vi "MGI Set Table Scrollbar.vi"(10 "Error In":errorcluster, 11 "Listbox Reference In":refnum<vi>) -> (2 "Error Out":errorcluster, 3 "Listbox Reference Out":refnum<vi>)   [LabVIEW 2020]
doc: "Show or hide the specified Table's horizontal and vertical scrollbars based on the table's contents. This VI will also set the scrollbar position as necessary to ensure that some of the table's contents is displayed.\n\nAuthored by Shawn Walpole\nsupport@mooregoodideas.com\nwww.mooregoodideas.com\n\nCopyright (c) 2010, Moore Good Ideas, Inc.\n\nAll rights reserved.\n\nRedistribution and use in source and binary forms, with or without modification, are permitted provided that the following conditions are met:\n\n * Redistributions of source code must retain the above copyright notice, this list of conditions and the following disclaimer.\n * Redistributions in binary form must reproduce the above copyright notice, this list of conditions and the following disclaimer in the documentation and/or other materials provided with the distribution.\n * Neither the name of Moore Good Ideas, Inc. nor the names of its contributors may be used to endorse or promote products derived from this software without specific prior written permission.\n\nTHIS SOFTWARE IS PROVIDED BY THE COPYRIGHT HOLDERS AND CONTRIBUTORS \"AS IS\" AND ANY EXPRESS OR IMPLIED WARRANTIES, INCLUDING, BUT NOT LIMITED TO, THE IMPLIED WARRANTIES OF MERCHANTABILITY AND FITNESS FOR A PARTICULAR PURPOSE ARE DISCLAIMED. IN NO EVENT SHALL THE COPYRIGHT OWNER OR CONTRIBUTORS BE LIABLE FOR ANY DIRECT, INDIRECT, INCIDENTAL, SPECIAL, EXEMPLARY, OR CONSEQUENTIAL DAMAGES (INCLUDING, BUT NOT LIMITED TO, PROCUREMENT OF SUBSTITUTE GOODS OR SERVICES; LOSS OF USE, DATA, OR PROFITS; OR BUSINESS INTERRUPTION) HOWEVER CAUSED AND ON ANY THEORY OF LIABILITY, WHETHER IN CONTRACT, STRICT LIABILITY, OR TORT (INCLUDING NEGLIGENCE OR OTHERWISE) ARISING IN ANY WAY OUT OF THE USE OF THIS SOFTWARE, EVEN IF ADVISED OF THE POSSIBILITY OF SUCH DAMAGE."
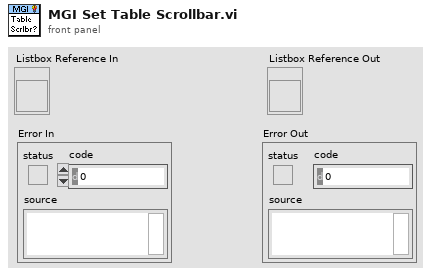
[diagram p1: front panel]
types:
  T1 = typedef "LVRowAndColumnUnsignedTypeDef.ctl" = cluster{"Row":u32, "Column":u32}
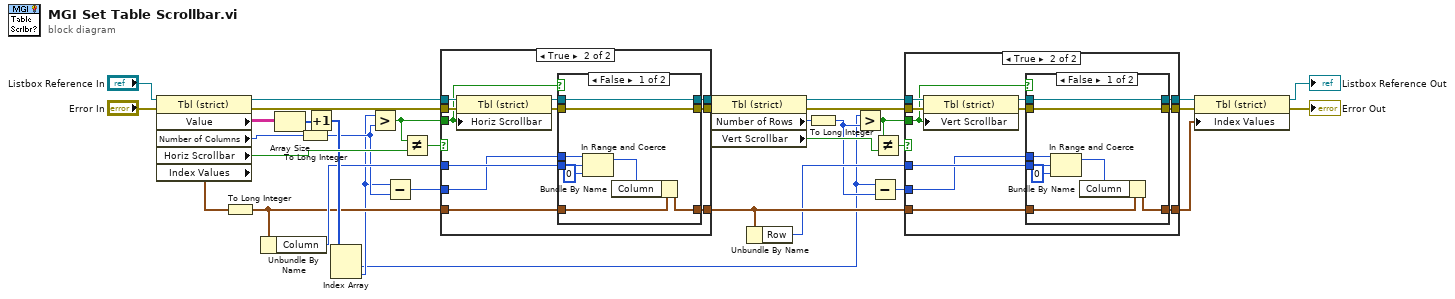
[diagram p0: block diagram]
diagram:
  n1 = property class="Tbl (strict)"(reference="Listbox Reference In", error in="Error In") -> (reference out=w35:refnum<vi>, error out=w27:errorcluster, "Value"=w33:string[][], "Number of Columns"=w26:u32, "Horiz Scrollbar"=w31:bool, "Index Values"=w6:T1)
  n2 = To Long Integer(number=w6) -> (32bit integer=w5:cluster{"Row":i32, "Column":i32})
  n3 = Unbundle By Name(w5) -> ("Column"=w23:i32)
  n4 = Array Size(array=w33) -> (size(s)=w32:i32[])
  n5 = To Long Integer(number=w26) -> (32bit integer=w7:i32)
  n6 = Increment(x=w32) -> (x+1=w24:i32[])
  n7 = Index Array(array=w24) -> (element #1=w1:i32, element #2=w2:i32)  [unwired: 2 in]
  n8 = Greater?(x=w2, y=w7) -> (0:w30:bool)
  n9 = Subtract(x=w2, y=w7) -> (x-y=w25:i32)
  n10 = Not Equal?(x=w30, y=w31) -> (x != y?=w29:bool)
  n11 = case shown="True" w29 {
    tunnel: w35 -> [w38 w49]
    tunnel: w30 -> [_ w43]
    tunnel: [w38 w45] -> w18
    tunnel: w27 -> [w37 w48]
    tunnel: [w37 w44] -> w16
    tunnel: w23 -> [_ w42]
    tunnel: w25 -> [_ w41]
    tunnel: w5 -> [w36 w40]
    tunnel: [w36 w39] -> w20
    frame False {
    }
    frame True {
      n12 = property class="Tbl (strict)"(reference=w49, error in=w48, "Horiz Scrollbar"=w43) -> (reference out=w47:refnum<vi>, error out=w46:errorcluster)
      n13 = case shown="False" w43 {
        tunnel: w47 -> [w52 w60]
        tunnel: w46 -> [w53 w59]
        tunnel: [w52 w60] -> w45
        tunnel: [w53 w59] -> w44
        tunnel: w42 -> [w57 _]
        tunnel: w41 -> [w55 _]
        tunnel: w40 -> [w54 w58]
        tunnel: [w50 w58] -> w39
        frame False {
          n14 = In Range and Coerce(upper limit=w55, x=w57, lower limit=0) -> (coerced(x)=w51:i32)  [unwired: 1 out]
          n15 = Bundle By Name(cluster=w54, "Column"=w51) -> (w50:cluster{"Row":i32, "Column":i32})
        }
        frame True {
        }
      }
    }
  }
  n16 = property class="Tbl (strict)"(reference=w18, error in=w16) -> (reference out=w19:refnum<vi>, error out=w17:errorcluster, "Number of Rows"=w4:u32, "Vert Scrollbar"=w14:bool)
  n17 = Unbundle By Name(w20) -> ("Row"=w15:i32)
  n18 = To Long Integer(number=w4) -> (32bit integer=w3:i32)
  n19 = Greater?(x=w1, y=w3) -> (0:w13:bool)
  n20 = Subtract(x=w1, y=w3) -> (x-y=w21:i32)
  n21 = Not Equal?(x=w13, y=w14) -> (x != y?=w22:bool)
  n22 = case shown="True" w22 {
    tunnel: w19 -> [w63 w74]
    tunnel: w13 -> [_ w68]
    tunnel: [w63 w70] -> w9
    tunnel: w17 -> [w62 w73]
    tunnel: [w62 w69] -> w10
    tunnel: w15 -> [_ w67]
    tunnel: w21 -> [_ w66]
    tunnel: w20 -> [w61 w65]
    tunnel: [w61 w64] -> w8
    frame False {
    }
    frame True {
      n23 = property class="Tbl (strict)"(reference=w74, error in=w73, "Vert Scrollbar"=w68) -> (reference out=w72:refnum<vi>, error out=w71:errorcluster)
      n24 = case shown="False" w68 {
        tunnel: w72 -> [w77 w85]
        tunnel: w71 -> [w78 w84]
        tunnel: [w77 w85] -> w70
        tunnel: [w78 w84] -> w69
        tunnel: w67 -> [w82 _]
        tunnel: w66 -> [w80 _]
        tunnel: w65 -> [w79 w83]
        tunnel: [w75 w83] -> w64
        frame False {
          n25 = In Range and Coerce(upper limit=w80, x=w82, lower limit=0) -> (coerced(x)=w76:i32)  [unwired: 1 out]
          n26 = Bundle By Name(cluster=w79, "Column"=w76) -> (w75:cluster{"Row":i32, "Column":i32})
        }
        frame True {
        }
      }
    }
  }
  n27 = property class="Tbl (strict)"(reference=w9, error in=w10, "Index Values"=w8) -> (reference out=→"Listbox Reference Out":refnum<vi>, error out=→"Error Out":errorcluster)
